vi "Get SMO PGSQL Log Paths.vi"(5 "getAll Cluster":variant, 7 "Default Paths":string, 8 "error in (no error)":errorcluster, 11 "instrument.PPMS in":refnum<class "instrument.OptiCool.lvclass">) -> (0 "error out":errorcluster, 2 "Paths":string, 3 "instrument.PPMS out":refnum<class "instrument.OptiCool.lvclass">)   [LabVIEW 2019, in "instrument.OptiCool.lvclass"]
uses:
  instrument.OptiCool.lvclass
  instrument.PPMS/instrument.PPMS.lvclass
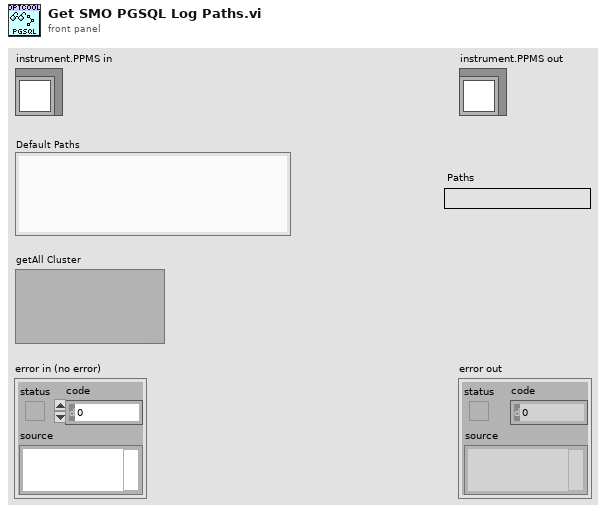
[diagram p1: front panel]
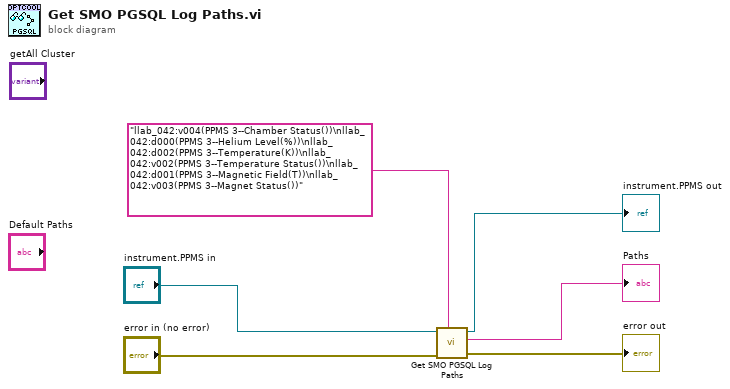
[diagram p0: block diagram]
diagram:
  n1 = call-parent "Get SMO PGSQL Log Paths.vi"("Default Paths"="llab_042:v004(PPMS 3--Chamber Status())\nllab_042:d000(PPMS 3--Helium Level(%))\nllab_042:d002(PPMS 3--Temperature(K))\nllab_042:v002(PPMS 3--Temperature Status())\nllab_042:d001(PPMS 3--Magnetic Field(T))\nllab_042:v003(PPMS 3--Magnet Status())" ("Paths"), "error in (no error)"="error in (no error)", "instrument.PPMS in"="instrument.PPMS in") -> ("error out"=→"error out":errorcluster, "Paths"=→"Paths":string, "instrument.PPMS out"=→"instrument.PPMS out":refnum<class "instrument.OptiCool.lvclass">)  [unwired: 6 in]
